vi "TB-Analyze.vi"(1 "state in":T2, 2 "persist":T1, 9 "AI Waveforms":dbl[][](array[numeric]), 11 "error in (no error)":errorcluster, 12 "Exposure parameters":T6={"Low cutoff (kHz)"=0.0, "High cutoff (kHz)"=0.0, "Duration (min)"=0.0, "dB SPL"=100.0, "Waveform"=enum."Noise", "WAVfile"=path "", "refWav"=path "", "use mic correction"=FALSE, "micCorrFile"=path "", "Pistonphone Level (dB SPL)"=0.0, "Sampling rate (Hz)"=0.0, "Buffer length (s)"=0.0, "Stream mic"=FALSE, "Fine adjust"={"Max"=0.0, "Min"=0.0}, "Mic gain"=0.0, "atten"=0.0, "Allow Slack"=FALSE, "max starts"=0, "Freq (kHz)"=8.0, "Tma (s)"=0.0, "Streamed"=[], "Drive"="", "Speaker"="", "Mic"="", "Analysis"={"Method"=enum."Default", "resol (Hz)"=0.0, "nfreq"=0, "signal"=""}, "exposeAtten"=0.0, "Digital"=""}, 13 "Pistonphone Factor":dbl) -> (3 "state out":T2, 4 "waveform":waveform(dbl), 6 "spectrum":waveform(dbl), 8 "Overload":bool, 10 "Cal SPL":dbl, 14 "history values":dbl[](array[numeric]), 15 "error out":errorcluster)   [LabVIEW 2020]
uses:
  Typedefs/TB-Parameters.ctl
  Typedefs/TB-Analysis Parameters.ctl
  Typedefs/TB-Runtime state.ctl
  <vilib>/sound2/lvsound2.llb/Sound File Refnum.ctl
  Typedefs/TB-Setup Log.ctl
  Typedefs/TB-Analysis State.ctl
  Typedefs/TB-Persistent Data.ctl
  <vilib>/Analysis/5stat.llb/RMS (DBL).vi
  7a26687d-8182-480d-aa8b-400f6e62ea30.vi
  a75af854-86a2-4979-89ec-6c460708d92b.vi
  24d8ff64-4411-4cbd-8f17-04fa62ccd382.vi
  5df69c7f-ca95-4c36-b998-4e8ba5f8752c.vi
  <vilib>/Analysis/baseanly.llb/Mean.vi
  <vilib>/Analysis/baseanly.llb/Mean (DBL).vi
  epl-vi-lib/Utility VIs/Math VIs/FFT x(t) to dB,Degrees (1D).vi
  <vilib>/Analysis/NI_AALPro.lvlib
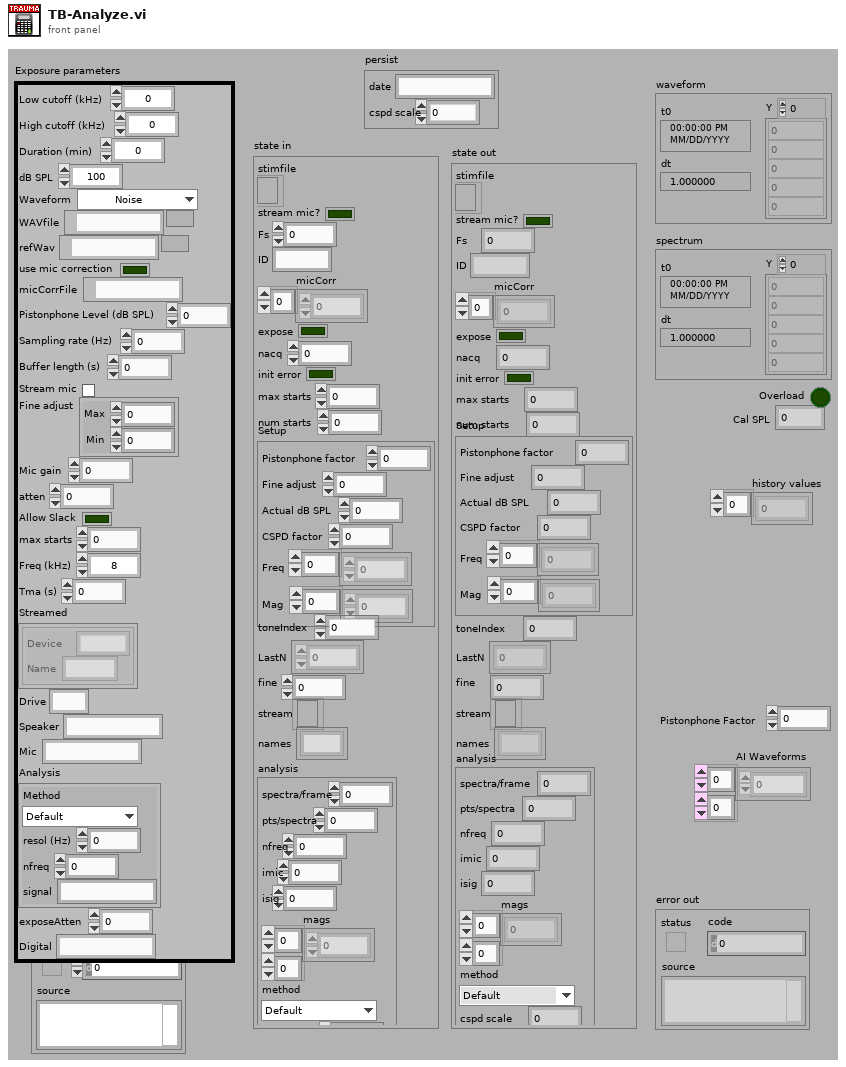
[diagram p1: front panel]
types:
  T1 = typedef "TB-Persistent Data.ctl" = cluster{"date":string, "cspd scale":dbl}
  T2 = typedef "TB-Runtime state.ctl" = cluster{"stimfile":T3, "stream mic?":bool, "Fs":dbl, "ID":string, "micCorr":dbl[], "expose":bool, "nacq":i32, "init error":bool, "max starts":i32, "num starts":i32, "Setup":T4, "toneIndex":i32, "LastN":dbl[], "fine":dbl, "stream":refnum<file>, "names":string[], "analysis":T5}
  T3 = typedef "Sound File Refnum.ctl" = refnum<file>
  T4 = typedef "TB-Setup Log.ctl" = cluster{"Pistonphone factor":dbl, "Fine adjust":dbl, "Actual dB SPL":dbl, "CSPD factor":dbl, "Freq":dbl[], "Mag":dbl[]}
  T5 = typedef "TB-Analysis State.ctl" = cluster{"spectra/frame":i32, "pts/spectra":i32, "nfreq":i32, "imic":i32, "isig":i32, "mags":dbl[][], "method":enum16{"Default", "Periodogram", "Cross-spectrum"}, "cspd scale":dbl}
  T6 = typedef "TB-Parameters.ctl" = cluster{"Low cutoff (kHz)":dbl, "High cutoff (kHz)":dbl, "Duration (min)":dbl, "dB SPL":dbl, "Waveform":enum16{"Noise", "File", "Tone"}, "WAVfile":path, "refWav":path, "use mic correction":bool, "micCorrFile":path, "Pistonphone Level (dB SPL)":dbl, "Sampling rate (Hz)":dbl, "Buffer length (s)":dbl, "Stream mic":bool, "Fine adjust":cluster{"Max":dbl, "Min":dbl}, "Mic gain":dbl, "atten":dbl, "Allow Slack":bool, "max starts":i32, "Freq (kHz)":dbl, "Tma (s)":dbl, "Streamed":cluster{"Device":string, "Name":string}[], "Drive":string, "Speaker":string, "Mic":string, "Analysis":T7, "exposeAtten":dbl, "Digital":string}
  T7 = typedef "TB-Analysis Parameters.ctl" = cluster{"Method":enum16{"Default", "Periodogram", "Cross-spectrum"}, "resol (Hz)":dbl, "nfreq":i32, "signal":string}
  T8 = enum16{"Default", "Periodogram", "Cross-spectrum"}
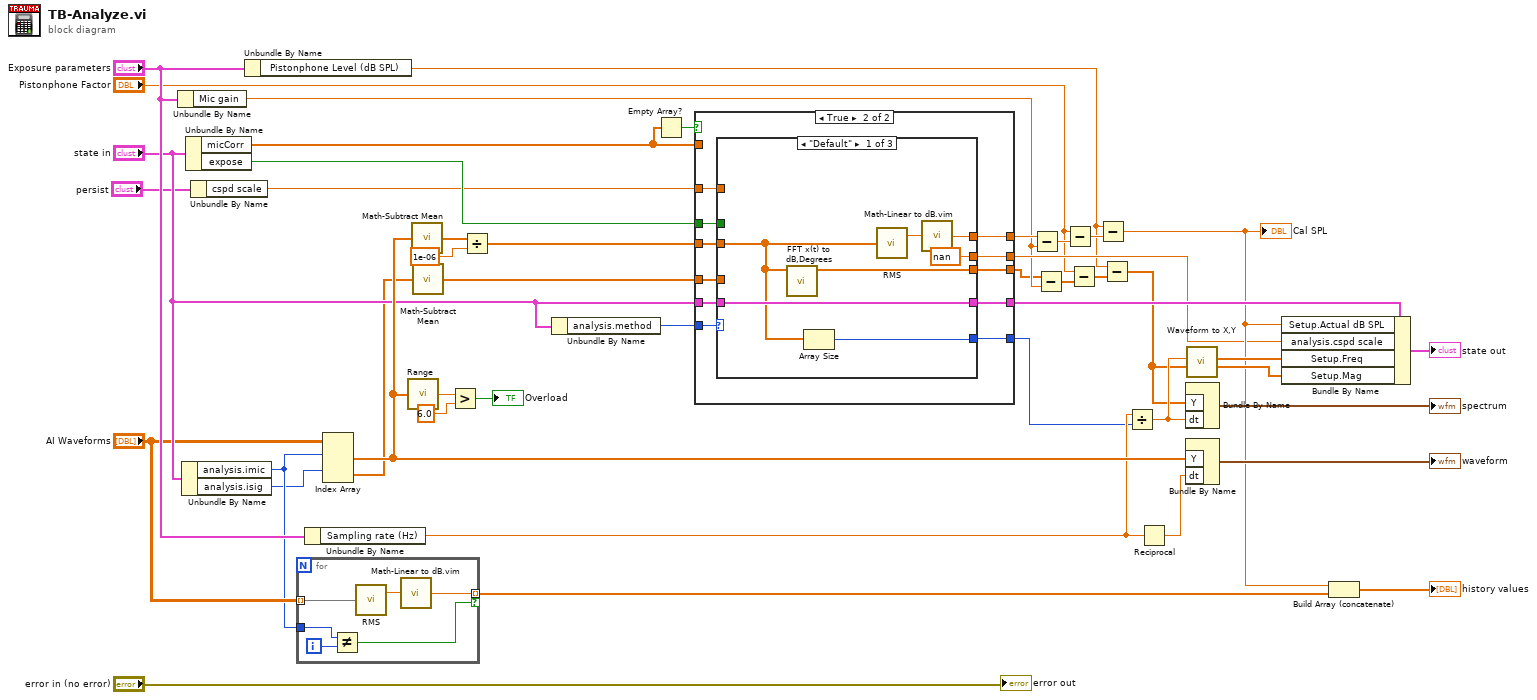
[diagram p0: block diagram]
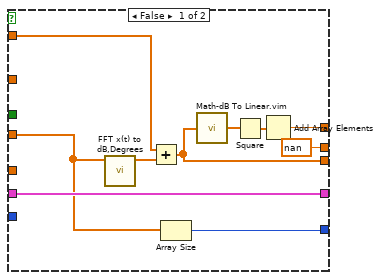
[diagram p2: hidden frame]
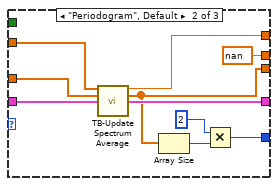
[diagram p3: hidden frame]
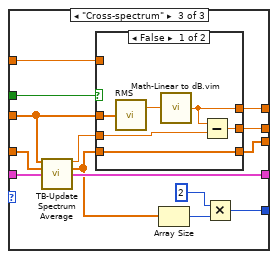
[diagram p4: hidden frame]
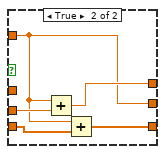
[diagram p5: hidden frame]
diagram:
  n1 = Unbundle By Name("Exposure parameters") -> ("Mic gain"=w5:dbl)
  n2 = Unbundle By Name("state in") -> ("analysis.imic"=w19:i32, "analysis.isig"=w15:i32)
  n3 = Unbundle By Name("state in") -> ("micCorr"=w27:dbl[], "expose"=w11:bool)
  n4 = Unbundle By Name("persist") -> ("cspd scale"=w9:dbl)
  n5 = Unbundle By Name("Exposure parameters") -> ("Pistonphone Level (dB SPL)"=w3:dbl)
  n6 = for {
    tunnel: "AI Waveforms" -> [w50] mode=indexing
    tunnel: [w49] -> w18 mode=indexing if=w46
    tunnel: w19 -> [w47]
    i -> [w48]
    n7 = Not Equal?(x=w47, y=w48) -> (x != y?=w46:bool)
    n8 = call-poly <vilib>:"RMS.vi"("X"=w50) -> ("rms value"=w51:dbl)  [unwired: 1 out]
    n9 = call "Math-Linear to dB.vim"("linear"=w51) -> ("dB"=w49:dbl)
  }
  n10 = Unbundle By Name("Exposure parameters") -> ("Sampling rate (Hz)"=w38:dbl)
  n11 = Index Array(array="AI Waveforms", index (row) #1=w19, index (row) #2=w15) -> (element #1=w42:dbl[], element #2=w14:dbl[])  [unwired: 2 in]
  n12 = call "Range.vi"("Array"=w42) -> ("Range"=w41:dbl)
  n13 = call "Math-Subtract Mean.vi"("Y"=w42) -> ("Y - mean(Y)"=w29:dbl[])  [unwired: 4 in]
  n14 = call "Math-Subtract Mean.vi"("Y"=w14) -> ("Y - mean(Y)"=w13:dbl[])  [unwired: 4 in]
  n15 = Greater?(x=w41, y=6.0) -> (0:→"Overload":bool)
  n16 = Divide(x=w29, y=1e-06) -> (x/y=w33:dbl[])
  n17 = Unbundle By Name("state in") -> ("analysis.method"=w12:T8)
  n18 = Empty Array?(array=w27) -> (empty?=w28:bool)
  n19 = case shown="True" w28 {
    tunnel: [w58 w72] -> w34
    tunnel: w33 -> [w53 w71]
    tunnel: w27 -> [w57 _]
    tunnel: [w61 w70] -> w2
    tunnel: "state in" -> [w56 w69]
    tunnel: [w56 w68] -> w32
    tunnel: [w55 w67] -> w30
    tunnel: w13 -> [_ w66]
    tunnel: w12 -> [_ w65]
    tunnel: w11 -> [_ w64]
    tunnel: w9 -> [_ w63]
    tunnel: [nan ("cspd scale") w62] -> w8
    frame False {
      n20 = call-poly "FFT x(t) to dB,Degrees.vi"("X"=w53) -> ("+Freq. Mag of FFT (dB rms)"=w54:dbl[])  [unwired: 8 in, 2 out]
      n21 = Add(x=w57, y=w54) -> (x+y=w61:dbl[])
      n22 = Array Size(array=w53) -> (size(s)=w55:i32)
      n23 = call "Math-dB To Linear.vim"("dB"=w61) -> ("linear"=w59:dbl[])
      n24 = Square(x=w59) -> (x^2=w60:dbl[])
      n25 = Add Array Elements(numeric array=w60) -> (sum=w58:dbl)
    }
    frame True {
      n26 = case shown="\"Default\"" w65 {
        tunnel: [w79 w89 w95] -> w72
        tunnel: w71 -> [w75 w82 w96]
        tunnel: [w74 w86 w90] -> w70
        tunnel: w69 -> [w77 w87 w102]
        tunnel: [w77 w88 w103] -> w68
        tunnel: [w76 w83 w99] -> w67
        tunnel: w66 -> [_ w81 w98]
        tunnel: w64 -> [_ _ w97]
        tunnel: w63 -> [_ _ w93]
        tunnel: [nan ("cspd scale") nan ("cspd scale") w92] -> w62
        frame "Default" {
          n27 = call-poly "FFT x(t) to dB,Degrees.vi"("X"=w75) -> ("+Freq. Mag of FFT (dB rms)"=w74:dbl[])  [unwired: 8 in, 2 out]
          n28 = Array Size(array=w75) -> (size(s)=w76:i32)
          n29 = call-poly <vilib>:"RMS.vi"("X"=w75) -> ("rms value"=w78:dbl)  [unwired: 1 out]
          n30 = call "Math-Linear to dB.vim"("linear"=w78) -> ("dB"=w79:dbl)
        }
        frame "Periodogram", Default {
          n31 = call "TB-Update Spectrum Average.vi"("mic"=w82, "stim"=w81, "state in"=w87) -> ("RMS"=w89:dbl, "Mag"=w86:dbl[], "state out"=w88:T2)  [unwired: 10 in]
          n32 = Array Size(array=w86) -> (size(s)=w85:i32)
          n33 = Multiply(x=2, y=w85) -> (x*y=w83:i32)
        }
        frame "Cross-spectrum" {
          n34 = call "TB-Update Spectrum Average.vi"("mic"=w96, "stim"=w98, "state in"=w102) -> ("RMS"=w94:dbl, "Mag"=w91:dbl[], "state out"=w103:T2)  [unwired: 10 in]
          n35 = case shown="False" w97 {
            tunnel: w96 -> [w108 _]
            tunnel: [w107 w113] -> w95
            tunnel: w94 -> [w106 w114]
            tunnel: w93 -> [_ w112]
            tunnel: [w105 w112] -> w92
            tunnel: w91 -> [w104 w111]
            tunnel: [w104 w110] -> w90
            frame False {
              n36 = call-poly <vilib>:"RMS.vi"("X"=w108) -> ("rms value"=w109:dbl)  [unwired: 1 out]
              n37 = call "Math-Linear to dB.vim"("linear"=w109) -> ("dB"=w107:dbl)
              n38 = Subtract(x=w107, y=w106) -> (x-y=w105:dbl)
            }
            frame True {
              n39 = Add(x=w112, y=w114) -> (x+y=w113:dbl)
              n40 = Add(x=w112, y=w111) -> (x+y=w110:dbl[])
            }
          }
          n41 = Array Size(array=w91) -> (size(s)=w101:i32)
          n42 = Multiply(x=2, y=w101) -> (x*y=w99:i32)
        }
      }
    }
  }
  n43 = Subtract(x=w34, y=w5) -> (x-y=w36:dbl)
  n44 = Subtract(x=w2, y=w5) -> (x-y=w6:dbl[])
  n45 = Subtract(x="Pistonphone Factor", y=w36) -> (x-y=w37:dbl)
  n46 = Subtract(x="Pistonphone Factor", y=w6) -> (x-y=w7:dbl[])
  n47 = Subtract(x=w3, y=w37) -> (x-y=w16:dbl)
  "Cal SPL" <- w16
  n48 = Subtract(x=w3, y=w7) -> (x-y=w1:dbl[])
  n49 = Divide(x=w38, y=w30) -> (x/y=w22:dbl)
  n50 = Reciprocal(x=w38) -> (1/x=w44:dbl)
  n51 = Bundle By Name("Y"=w1, "dt"=w22) -> (→"spectrum":waveform(dbl))  [unwired: 1 in]
  n52 = Bundle By Name("Y"=w42, "dt"=w44) -> (→"waveform":waveform(dbl))  [unwired: 1 in]
  n53 = call "Waveform to X,Y.vi"("Y"=w1, "dx"=w22) -> ("Y"=w23:dbl[], "X"=w24:dbl[])  [unwired: 5 in]
  n54 = Bundle By Name(cluster=w32, "Setup.Actual dB SPL"=w16, "analysis.cspd scale"=w8, "Setup.Freq"=w24, "Setup.Mag"=w23) -> (→"state out":T2)
  n55 = Build Array (concatenate)(w16, w18) -> (→"history values":dbl[])
  "error out" <- "error in (no error)"
